vi "setRange.vi"(8 "error in (no error)":errorcluster, 10 "Range":cluster{"units":string, "min":dbl, "max":dbl}, 11 "AnalogDevice.lvclass in":refnum<class "AnalogDevice.lvclass">) -> (0 "error out":errorcluster, 3 "AnalogDevice.lvclass out":refnum<class "AnalogDevice.lvclass">)   [LabVIEW 2009, in "Tools.lvlib" / "DatabaseHelpers.lvlib" / "AnalogDevice.lvclass"]
uses:
  AnalogDevice.lvclass
  AnalogDevice.lvclass/AnalogDevice.ctl
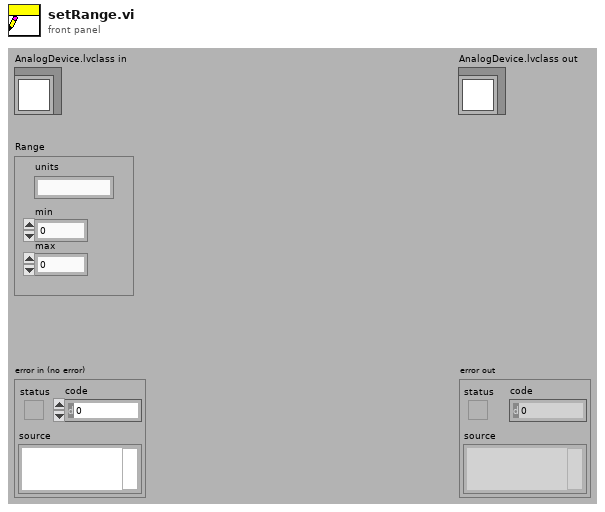
[diagram p1: front panel]
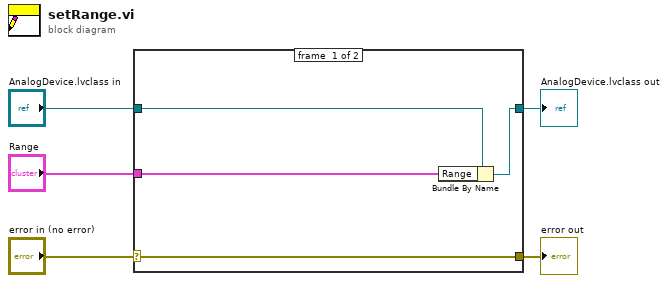
[diagram p0: block diagram]
diagram:
  n1 = case shown="No Error" "error in (no error)" {
    selector: "error in (no error)" -> [w9 w10]
    tunnel: [w9 w10] -> w4
    tunnel: [w7 w11] -> w2
    tunnel: "AnalogDevice.lvclass in" -> [w8 w11]
    tunnel: "Range" -> [w6 _]
    frame #0 {
      n2 = Bundle By Name(cluster=w8, "Range"=w6) -> (w7:refnum<class "AnalogDevice.lvclass">)
    }
    frame #1 {
    }
  }
  "error out" <- w4
  "AnalogDevice.lvclass out" <- w2
